vi "Start.vi"(8 "error in (no error)":errorcluster, 10 "Active?":bool) -> (0 "error out":errorcluster, 3 "Speedometer out":refnum<class "Speedometer.lvclass">)   [LabVIEW 2026, in "TALOS.lvlib" / "Classes.lvlib" / "Speedometer.lvclass"]
uses:
  Speedometer.lvclass
  Speedometer.lvclass/Speedometer.ctl
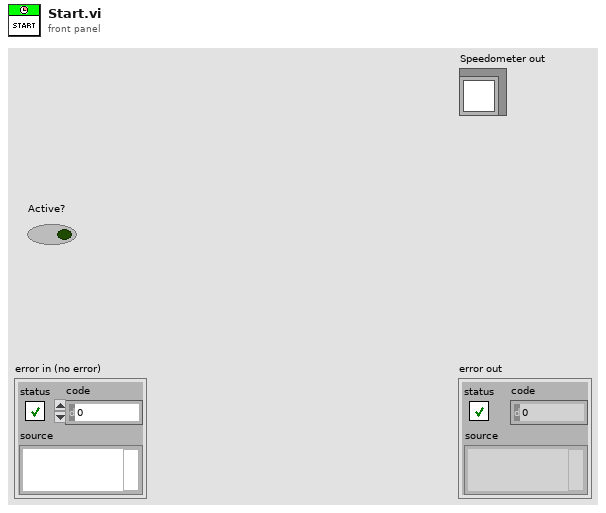
[diagram p1: front panel]
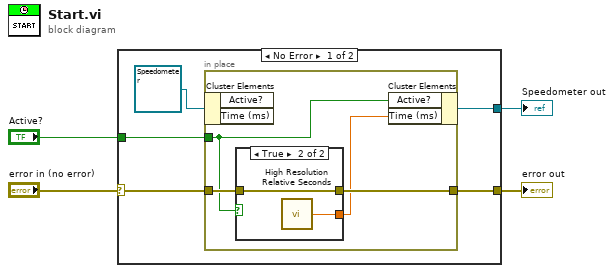
[diagram p0: block diagram]
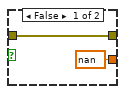
[diagram p2: hidden frame]
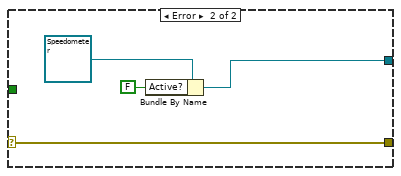
[diagram p3: hidden frame]
diagram:
  n1 = case shown="No Error" "error in (no error)" {
    selector: "error in (no error)" -> [w5 w21]
    tunnel: [w9 w21] -> w3
    tunnel: [w8 w18] -> w2
    tunnel: "Active?" -> [w6 _]
    frame No Error {
      n2 = in-place {
        in-place-border: w5 -> [w13]
        in-place-border: [w12] -> w9
        in-place-border: w6 -> [w10]
        n3 = in-place-cluster #1(refnum<class "Speedometer.lvclass"> refnum ("Speedometer in")) -> ()  [unwired: 2 out]
        n4 = case shown="True" w10 {
          tunnel: [w15 w17] -> w12
          tunnel: w13 -> [w15 w17]
          tunnel: [nan ("relative seconds") w16] -> w11
          frame False {
          }
          frame True {
            n5 = call <vilib>:"High Resolution Relative Seconds.vi"() -> ("relative seconds"=w16:dbl)
          }
        }
        n6 = in-place-cluster #1("Active?"=w10, "Time (ms)"=w11) -> (w8:refnum<class "Speedometer.lvclass">)
      }
    }
    frame Error {
      n7 = Bundle By Name(cluster=refnum<class "Speedometer.lvclass"> refnum ("Speedometer in"), "Active?"=FALSE) -> (w18:refnum<class "Speedometer.lvclass">)
    }
  }
  "error out" <- w3
  "Speedometer out" <- w2
